vi "Histogram Main.vi"() -> ()   [LabVIEW 2015]
uses:
  Consumer Message.ctl
  <vilib>/ErrorRing/Error Ring.xnode
panel:
  out "XY Graph":cluster{"X":dbl, "Y":dbl}[](graph)
  in  "bins":i32=20
  in  "signal":u16(ring) items=["uniform white", "uniform+uniform", "Gaussian white", "sine", "square"]
  out "Consumer Shutdown?":bool
  out "State to Execute":string
  out "High Priority?":bool
  out "Backlog":u8(slide) scale=0.0..100.0
  out "Processed Value":i32
  in  "High Priority Message":bool
  in  "Normal Priority Message":bool
  in  "Stop":bool
  # "Number of enqueued messages waiting to be processed"
  # "Current data being processed in consumer loop"
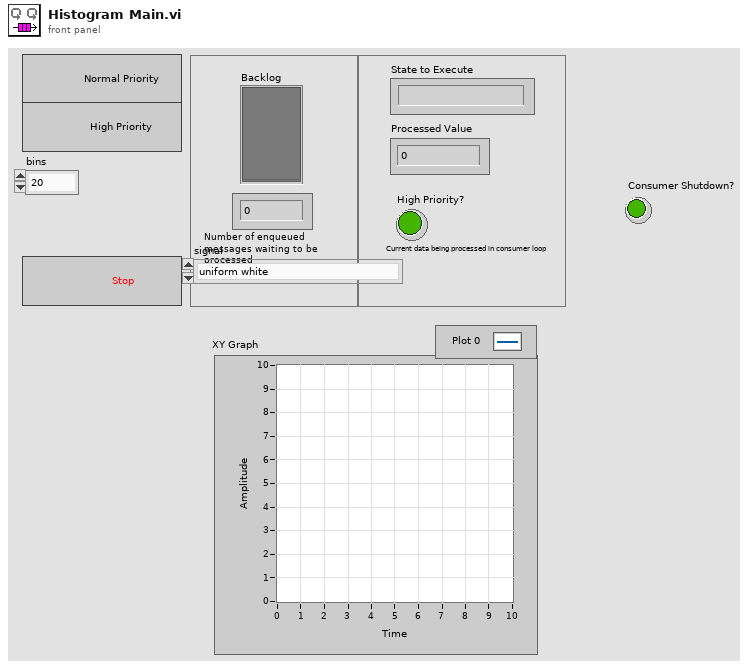
[diagram p1: front panel]
types:
  T1 = typedef "Consumer Message.ctl" = cluster{"Consumer State":string, "Boolean Data":bool, "Numeric Data":i32, "Signal":dbl[], "Error":errorcluster}
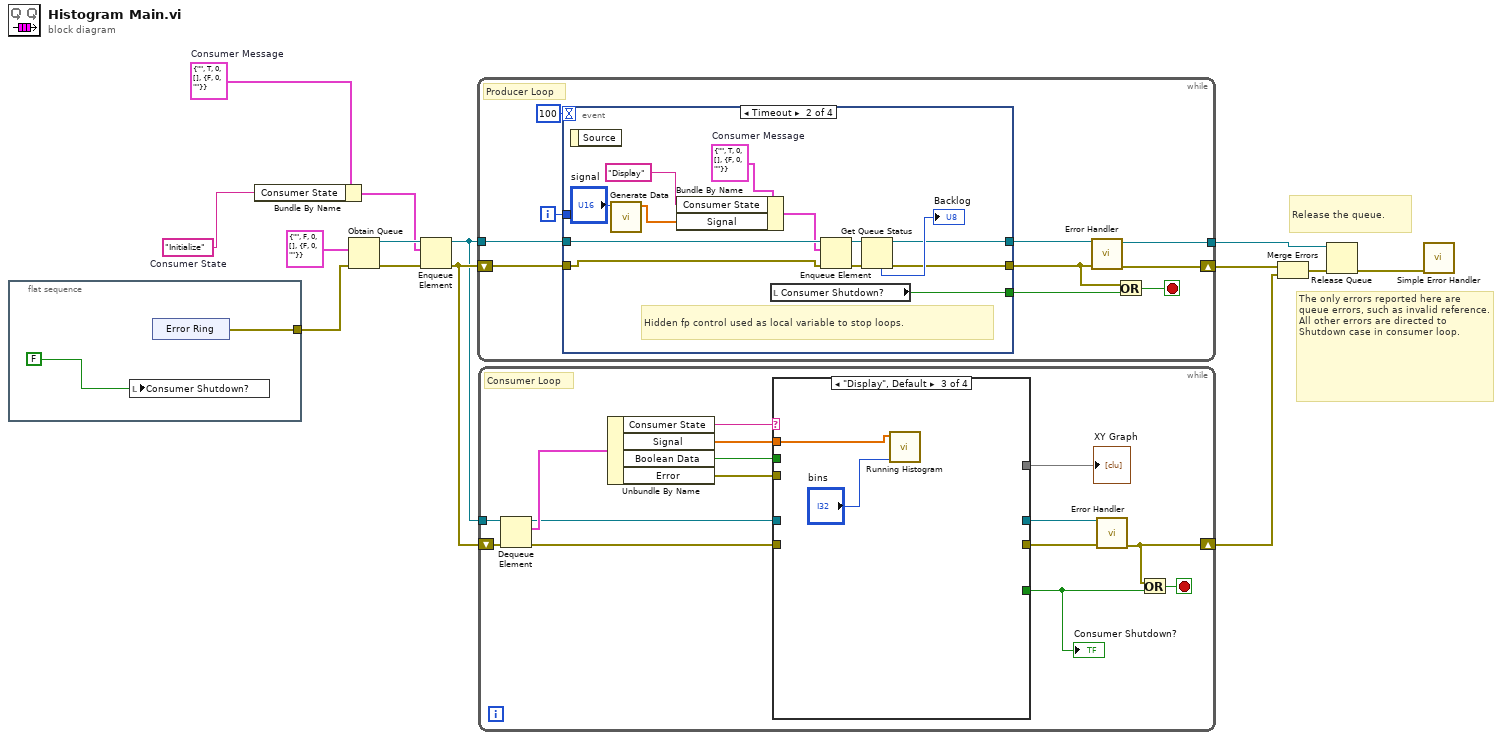
[diagram p0: block diagram]
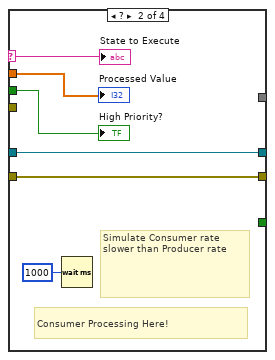
[diagram p3: hidden frame]
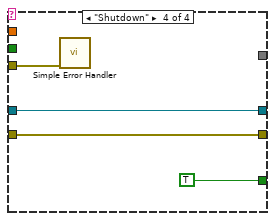
[diagram p4: hidden frame]
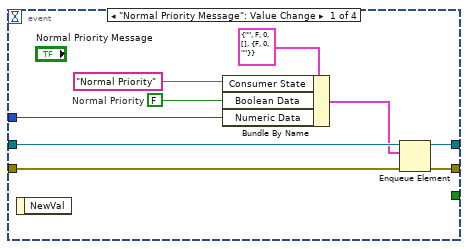
[diagram p5: hidden frame]
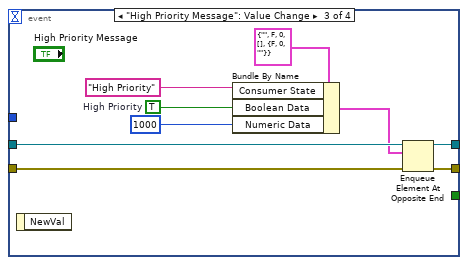
[diagram p6: hidden frame]
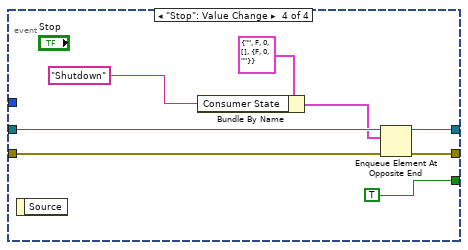
[diagram p7: hidden frame]
diagram:
  w6 = "Initialize"  # Consumer State
  w8 = T1 {"Consumer State"="", "Boolean Data"=TRUE, "Numeric Data"=0, "Signal"=[], "Error"={"status"=FALSE, "code"=0, "source"=""}}  # Consumer Message
  # "Release the queue."
  # "The only errors reported here are queue errors, such as invalid reference.  All other errors are directed to Shutdown case in consumer loop."
  n1 = flat-sequence {
    tunnel: [w15] -> w9
    frame #0 {
      n2 = local write "Consumer Shutdown?"(FALSE ("Stop Loops (local)")) -> ()
      n3 = xnode "Error Ring"() -> ("error out"=w15:errorcluster)
    }
  }
  n4 = Bundle By Name(cluster=w8, "Consumer State"=w6) -> (w7:T1)
  n5 = Obtain Queue(element data type=T1 {"Consumer State"="", "Boolean Data"=FALSE, "Numeric Data"=0, "Signal"=[], "Error"={"status"=FALSE, "code"=0, "source"=""}}, error in (no error)=w9) -> (queue out=w11:refnum<queue>, error out=w14:errorcluster)  [unwired: 3 in, 1 out]
  n6 = Enqueue Element(queue=w11, element=w7, error in (no error)=w14) -> (queue out=w10:refnum<queue>, error out=w12:errorcluster)  [unwired: 1 in, 1 out]
  n7 = while {
    tunnel: w10 -> [w27]
    shift-right: [w19] -> w5
    shift-left: w12 -> [w26]
    tunnel: [w18] -> w1
    i -> [w25]
    stop <- w21 stop-if-true
    # "Producer Loop"
    n8 = event shown="[1] Timeout" {
      selector: _ -> [_ _ _ _]
      dyn-events: _ -> [_ _ _ _]
      timeout: 100 -> [_ _ _ _]
      tunnel: w27 -> [w36 w47 w57 w66]
      tunnel: w26 -> [w34 w37 w56 w64]
      tunnel: [w35 w46 w58 w63] -> w20
      tunnel: [_ w49 _ TRUE] -> w22
      tunnel: w25 -> [w33 _ _ _]
      tunnel: [w29 w45 w52 w62] -> w24
      event "Normal Priority Message": Value Change {
        w30 = FALSE  # Normal Priority
        n9 = event-data() -> ()  [unwired: 1 in, 1 out]
        n10 = Bundle By Name(cluster=T1 {"Consumer State"="", "Boolean Data"=FALSE, "Numeric Data"=0, "Signal"=[], "Error"={"status"=FALSE, "code"=0, "source"=""}}, "Consumer State"="Normal Priority" ("String Data"), "Boolean Data"=w30, "Numeric Data"=w33) -> (w32:T1)
        n11 = Enqueue Element(queue=w36, element=w32, error in (no error)=w34) -> (queue out=w29:refnum<queue>, error out=w35:errorcluster)  [unwired: 1 in, 1 out]
      }
      event Timeout {
        w44 = T1 {"Consumer State"="", "Boolean Data"=TRUE, "Numeric Data"=0, "Signal"=[], "Error"={"status"=FALSE, "code"=0, "source"=""}}  # Consumer Message
        # "Hidden fp control used as local variable to stop loops."
        n12 = event-data() -> ()  [unwired: 1 in, 1 out]
        n13 = call "Generate Data.vi"("signal"="signal") -> ("Y"=w42:dbl[])  [unwired: 9 in, 1 out]
        n14 = Bundle By Name(cluster=w44, "Consumer State"="Display", "Signal"=w42) -> (w39:T1)
        n15 = local read "Consumer Shutdown?"() -> (w49:bool)
        n16 = Enqueue Element(queue=w47, element=w39, error in (no error)=w37) -> (queue out=w40:refnum<queue>, error out=w38:errorcluster)  [unwired: 1 in, 1 out]
        n17 = Get Queue Status(queue=w40, error in (no error)=w38) -> (queue out=w45:refnum<queue>, error out=w46:errorcluster, # elements in queue=→"Backlog":i32)  [unwired: 1 in, 5 out]
      }
      event "High Priority Message": Value Change {
        w51 = TRUE  # High Priority
        n18 = event-data() -> ()  [unwired: 1 in, 1 out]
        n19 = Bundle By Name(cluster=T1 {"Consumer State"="", "Boolean Data"=FALSE, "Numeric Data"=0, "Signal"=[], "Error"={"status"=FALSE, "code"=0, "source"=""}}, "Consumer State"="High Priority" ("String Data"), "Boolean Data"=w51, "Numeric Data"=1000) -> (w54:T1)
        n20 = Enqueue Element At Opposite End(queue=w57, element=w54, error in (no error)=w56) -> (queue out=w52:refnum<queue>, error out=w58:errorcluster)  [unwired: 1 in, 1 out]
      }
      event "Stop": Value Change {
        n21 = event-data() -> ()  [unwired: 1 in, 1 out]
        n22 = Bundle By Name(cluster=T1 {"Consumer State"="", "Boolean Data"=FALSE, "Numeric Data"=0, "Signal"=[], "Error"={"status"=FALSE, "code"=0, "source"=""}}, "Consumer State"="Shutdown") -> (w59:T1)
        n23 = Enqueue Element At Opposite End(queue=w66, element=w59, error in (no error)=w64) -> (queue out=w62:refnum<queue>, error out=w63:errorcluster)  [unwired: 1 in, 1 out]
      }
    }
    n24 = call "Error Handler.vi"("error in"=w20, "queue in"=w24) -> ("error out"=w19:errorcluster, "queue out"=w18:refnum<queue>)  [unwired: 8 in]
    n25 = Or(x=w20, y=w22) -> (x .or. y?=w21:bool)
  }
  n26 = while {
    tunnel: w10 -> [w81]
    shift-right: [w70] -> w4
    shift-left: w12 -> [w80]
    stop <- w71 stop-if-true
    # "Consumer Loop"
    n27 = Dequeue Element(queue=w81, error in (no error)=w80) -> (queue out=w69:refnum<queue>, element=w79:T1, error out=w68:errorcluster)  [unwired: 1 in, 1 out]
    n28 = Unbundle By Name(w79) -> ("Consumer State"=w78:string, "Signal"=w77:dbl[], "Boolean Data"=w76:bool, "Error"=w73:errorcluster)
    n29 = case shown="\"Display\", Default" w78 {
      selector: w78 -> [_ w86 _ _]
      tunnel: [_ _ _ TRUE] -> w72
      tunnel: w68 -> [w82 w84 _ w92]
      tunnel: [w82 w84 _ w92] -> w75
      tunnel: w77 -> [_ w89 w91 _]
      tunnel: w76 -> [_ w88 _ _]
      tunnel: w69 -> [w83 w87 _ w93]
      tunnel: [w83 w87 _ w93] -> w74
      tunnel: w73 -> [_ _ _ w94]
      tunnel: [_ _ _ _] -> w67
      frame "Initialize" {
      }
      frame ? {
        # "Simulate Consumer rate slower than Producer rate"
        # "Consumer Processing Here!"
        n30 = Wait (ms)(milliseconds to wait=u32 1000) -> ()  [unwired: 1 out]
        "Processed Value" <- w89
        "High Priority?" <- w88
        "State to Execute" <- w86
      }
      frame "Display", Default {
        n31 = call "Running Histogram.vi"("bins"="bins", "input data"=w91) -> ()  [unwired: 6 in, 4 out]
      }
      frame "Shutdown" {
        n32 = call <vilib>:"Simple Error Handler.vi"("error in (no error)"=w94) -> ()  [unwired: 4 in, 5 out]
      }
    }
    "Consumer Shutdown?" <- w72
    "XY Graph" <- w67
    n33 = call "Error Handler.vi"("error in"=w75, "queue in"=w74) -> ("error out"=w70:errorcluster)  [unwired: 8 in, 1 out]
    n34 = Or(x=w70, y=w72) -> (x .or. y?=w71:bool)
  }
  n35 = Merge Errors(w5, w4) -> (w3:errorcluster)
  n36 = Release Queue(queue=w1, error in (no error)=w3) -> (error out=w2:errorcluster)  [unwired: 1 in, 2 out]
  n37 = call <vilib>:"Simple Error Handler.vi"("error in (no error)"=w2) -> ()  [unwired: 4 in, 5 out]
